vi "UTILITY Date String Days.vi"(8 "error in (no error)":errorcluster, 10 "First date":string="25/09/2005", 11 "Second date":string="25/09/2006") -> (0 "error out":errorcluster, 3 "Elapsed days":i32)   [LabVIEW 2019]
doc: "This VI outputs the number of elapsed days between two specified date strings. The VI converts the date strings to timestamps. It then uses those timestamps to calculate the number of elapsed days between the two dates."
panel:
  # "Select Help»Show Context Help and move the cursor \nover the VI icon to display help for this VI."
  # "Format: DD/MM/YY"
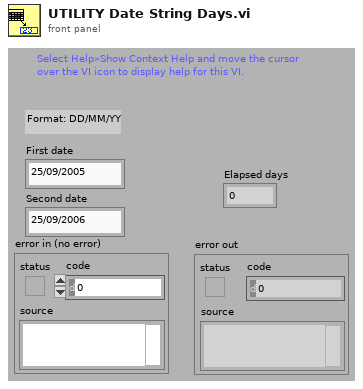
[diagram p1: front panel]
types:
  T1 = cluster{"fractional second":dbl, "second":i32, "minute":i32, "hour":i32, "day of month":i32, "month":i32, "year":i32, "day of week":i32, "day of year":i32, "DST":i32}
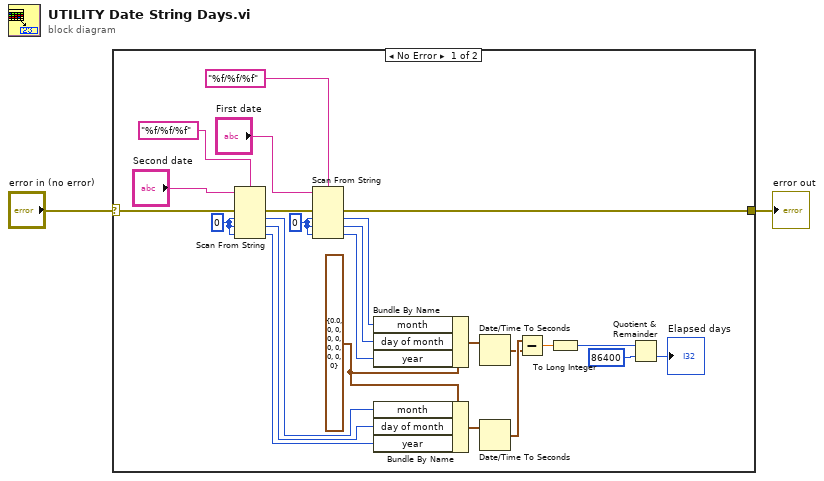
[diagram p0: block diagram]
diagram:
  n1 = case shown="No Error" "error in (no error)" {
    selector: "error in (no error)" -> [w5 w27]
    tunnel: [w6 w27] -> w1
    frame No Error {
      w10 = T1 {"fractional second"=0.0, "second"=0, "minute"=0, "hour"=0, "day of month"=0, "month"=0, "year"=0, "day of week"=0, "day of year"=0, "DST"=0} ("date time rec")
      w24 = 0
      w25 = 0
      n2 = Scan From String(format string="%f/%f/%f", input string="Second date", error in=w5, default 1=w25, default 2=w25, default 3=w25) -> (error out=w7:errorcluster, output 1=w20:i32, output 2=w19:i32, output 3=w18:i32)  [unwired: 1 in, 2 out]
      n3 = Scan From String(format string="%f/%f/%f", input string="First date", error in=w7, default 1=w24, default 2=w24, default 3=w24) -> (error out=w6:errorcluster, output 1=w17:i32, output 2=w16:i32, output 3=w15:i32)  [unwired: 1 in, 2 out]
      n4 = Bundle By Name(cluster=w10, "month"=w17, "day of month"=w16, "year"=w15) -> (w21:T1)
      n5 = Bundle By Name(cluster=w10, "month"=w20, "day of month"=w19, "year"=w18) -> (w22:T1)
      n6 = Date/Time To Seconds(2:w21) -> (0:w13:timestamp)  [unwired: 1 in]
      n7 = Date/Time To Seconds(2:w22) -> (0:w14:timestamp)  [unwired: 1 in]
      n8 = Subtract(x=w14, y=w13) -> (x-y=w12:dbl)
      n9 = To Long Integer(number=w12) -> (32bit integer=w8:i32)
      n10 = Quotient & Remainder(x=w8, y=86400) -> (floor(x/y)=→"Elapsed days":i32)  [unwired: 1 out]
    }
    frame Error {
    }
  }
  "error out" <- w1
